vi "test_Set Wait.vi"(8 "error in (no error)":errorcluster, 11 "Duration":u32 format="%.0x") -> (0 "error out":errorcluster, 3 "Data out":u64[](array[numeric])=[5631702913073631, 5629503829180420, 5629508124147720, 5629503829180426, 5629508124147722, 5629503829180426, 5629508124147722, 5629503829180426, 5629508124147722, 5631707147403291])   [LabVIEW 2016]
uses:
  Host/Typedefs/LV2G Operation.ctl
  Host/Typedefs/IO Buffer Operation.ctl
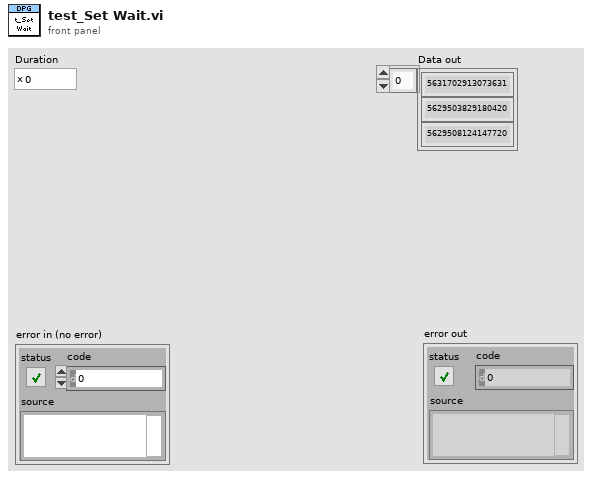
[diagram p1: front panel]
types:
  T1 = typedef "IO Buffer Operation.ctl" = enum16{"Initialize", "Write IO Data_Rd", "Read IO Data_Rd", "Write IO Data_Wr", "Read IO Data_Wr", "Write  IO Data_Dir", "Read  IO Data_Dir", "Write Host to Target FIFO", "Read Host to Target FIFO", "Write Target to Host FIFO", "Read Target to Host FIFO", "Write Monitor Enable?", "Read Monitor Enable?", "Close"}
  T2 = typedef "LV2G Operation.ctl" = enum16{"Initialize", "Set", "Get", "Close"}
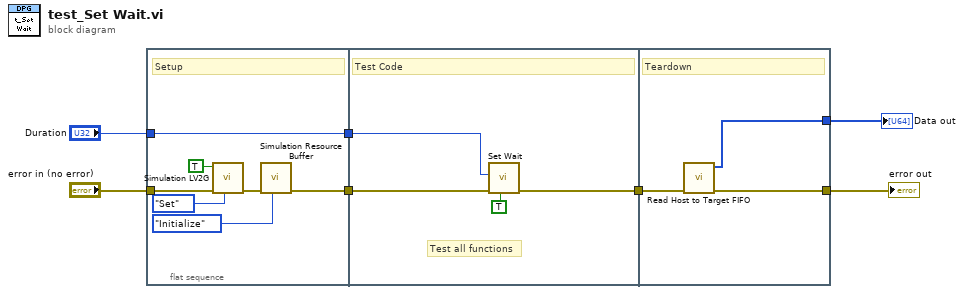
[diagram p0: block diagram]
diagram:
  n1 = flat-sequence {
    tunnel: "error in (no error)" -> [w14]
    tunnel: [w9] -> w7
    tunnel: "Duration" -> [w8]
    tunnel: [w8] -> w3
    tunnel: w7 -> [w18]
    tunnel: [w17] -> w6
    tunnel: w3 -> [w15]
    tunnel: [w20] -> w4
    tunnel: w6 -> [w21]
    tunnel: [w19] -> w2
    frame #0 {
      # "Setup"
      n2 = call "Simulation LV2G.vi"("Operation (Get)"=LV2G_Operation."Set", "error in (no error)"=w14, "Simulation?"=TRUE) -> ("error out"=w11:errorcluster)  [unwired: 7 in, 1 out]
      n3 = call "Simulation Resource Buffer.vi"("IO Buffer Operation"=IO_Buffer_Operation."Initialize", "error in (no error)"=w11) -> ("error out"=w9:errorcluster)  [unwired: 7 in, 2 out]
    }
    frame #1 {
      # "Test all functions"
      # "Test Code"
      n4 = call "Set Wait.vi"("Write to FPGA(T)"=TRUE, "error in (no error)"=w18, "Duration"=w15) -> ("error out"=w17:errorcluster)  [unwired: 7 in, 1 out]
    }
    frame #2 {
      # "Teardown"
      n5 = call "Read Host to Target FIFO.vi"("error in (no error)"=w21) -> ("error out"=w20:errorcluster, "Host to Target FIFO"=w19:u64[])  [unwired: 9 in]
    }
  }
  "error out" <- w4
  "Data out" <- w2
